vi "IsValidCoordinate.vi"(1 "Width":u32, 2 "Height":u32, 3 "Column":u32, 4 "Row":u32) -> (0 "Valid":bool)   [LabVIEW 2025]
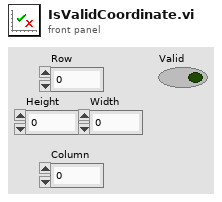
[diagram p1: front panel]
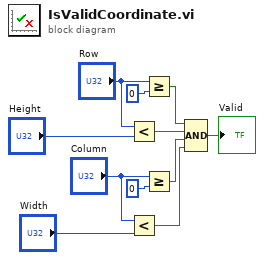
[diagram p0: block diagram]
diagram:
  n1 = Less?(x="Row", y="Height") -> (x < y?=w9:bool)
  n2 = Less?(x="Column", y="Width") -> (x < y?=w7:bool)
  n3 = Greater Or Equal?(x="Row", y=u32 0) -> (x >= y?=w10:bool)
  n4 = Greater Or Equal?(x="Column", y=u32 0) -> (x >= y?=w8:bool)
  n5 = Compound Arithmetic op=AND(w10, w9, w8, w7) -> (→"Valid":bool)
